vi "execute_value_write_policy.vi"(8 "error in (no error)":errorcluster, 9 "Publish Time":timestamp, 10 "New Topic Value":variant, 11 "OneShotSubscription In":refnum<class "OneShotSubscription.lvclass">) -> (0 "error out":errorcluster, 3 "OneShotSubscription Out":refnum<class "OneShotSubscription.lvclass">)   [LabVIEW 2017, in "SubscriptionPolicy.lvlib" / "OneShotSubscription.lvclass"]
uses:
  OneShotSubscription.lvclass
  C:/Git/mva-framework/Framework/IMediator/ISubscriptionPolicy/ISubscriptionPolicy.lvclass
  IMediator/ISubscriptionPolicy/ISubscriptionPolicy.lvclass/ISubscriptionPolicy.ctl
  <vilib>/Utility/error.llb/Error Cluster From Error Code.vi
  IMediator/ITransport/ITransport.lvclass
  <vilib>/ErrorRing/Error Ring.xnode
  IMediator/ISubscriptionPolicy/ISubscriptionPolicy.lvclass
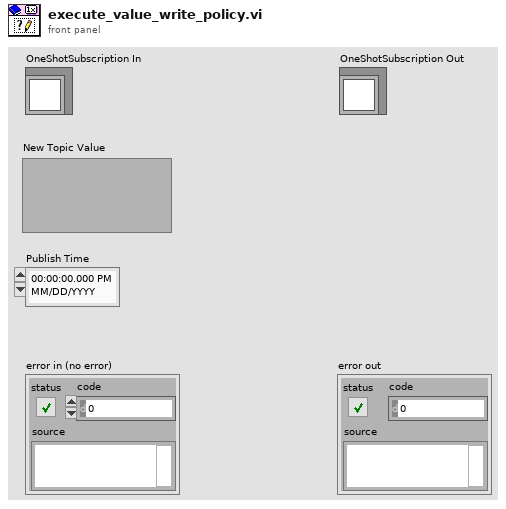
[diagram p1: front panel]
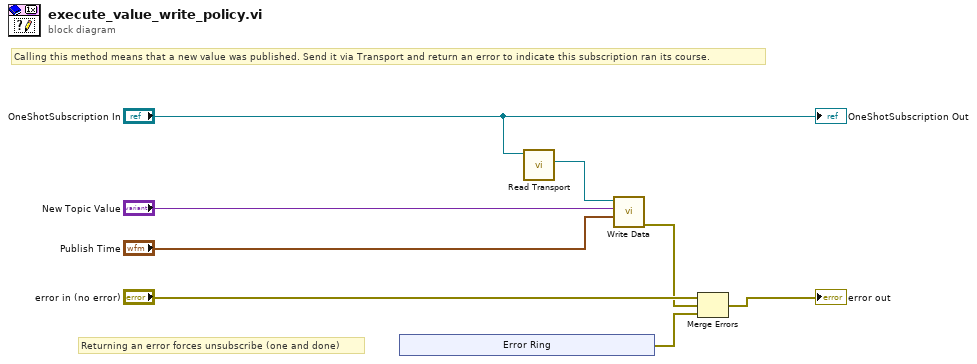
[diagram p0: block diagram]
diagram:
  # "Calling this method means that a new value was published. Send it via Transport and return an error to indicate this subscription ran its course."
  # "Returning an error forces unsubscribe (one and done)"
  n1 = xnode "Error Ring"() -> ("error out"=w2:errorcluster)
  n2 = call "Read Transport.vi"("ISubscriptionPolicy in"="OneShotSubscription In") -> ("Transport"=w3:refnum<class "ITransport.lvclass">)  [unwired: 10 in]
  n3 = call-dynamic "Write Data.vi"("Publication Time"="Publish Time", "Value"="New Topic Value", "ITransport in"=w3) -> ("error out"=w4:errorcluster)  [unwired: 7 in, 1 out]
  n4 = Merge Errors("error in (no error)", w4, w2) -> (→"error out":errorcluster)
  "OneShotSubscription Out" <- "OneShotSubscription In"
